vi "Ideal_Result_API.vi"(0 "Device DVR":refnum<data-value>, 11 "Error in":errorcluster) -> (4 "Device DVR":refnum<data-value>, 15 "Error Out":errorcluster)   [LabVIEW 2020, in "Device.lvclass"]
doc: "API to calculate Ideal Result"
uses:
  Device.lvclass
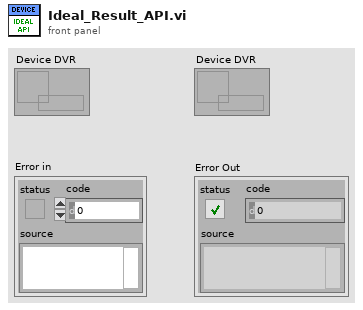
[diagram p1: front panel]
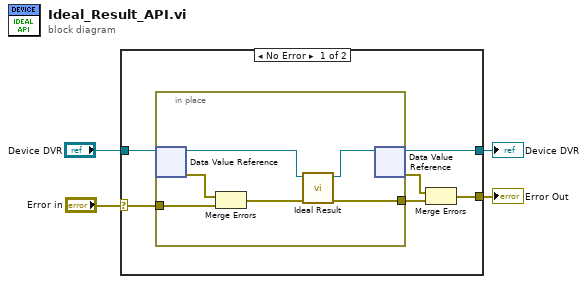
[diagram p0: block diagram]
diagram:
  n1 = case shown="No Error" "Error in" {
    selector: "Error in" -> [w9 w17]
    tunnel: "Device DVR" -> [w10 w18]
    tunnel: [w8 w18] -> w1
    tunnel: [w5 w17] -> w2
    frame No Error {
      n2 = in-place {
        in-place-border: w9 -> [w16]
        in-place-border: [w11] -> w7
        n3 = in-place-dvr #1(w10) -> (w13:refnum<class "Device.lvclass">, w15:errorcluster)
        n4 = Merge Errors(w15, w16) -> (w14:errorcluster)
        n5 = call-dynamic "Ideal Result.vi"("Error in"=w14, "Device in"=w13) -> ("Error out"=w11:errorcluster, "Device out"=w12:refnum<class "Device.lvclass">)  [unwired: 8 in]
        n6 = in-place-dvr #1(w12) -> (w8:refnum<data-value>, w6:errorcluster)
      }
      n7 = Merge Errors(w6, w7) -> (w5:errorcluster)
    }
    frame Error {
    }
  }
  "Error Out" <- w2
  "Device DVR" <- w1
